vi "Stop Producer LV2.vi"(0 "Stop":bool, 11 "Error In":errorcluster, 13 "Operation":T1) -> (4 "Stop":bool, 15 "Error Out":errorcluster)   [LabVIEW 2023]
doc: "The file is the functional global to store the status of the stop boolean which stops the producer loop."
uses:
  Typedef/User Event Operations.ctl
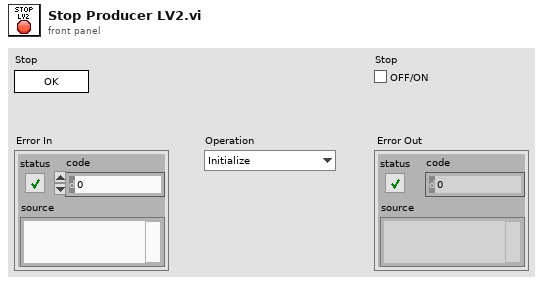
[diagram p1: front panel]
types:
  T1 = typedef "User Event Operations.ctl" = enum16{"Initialize", "Read", "Write"}
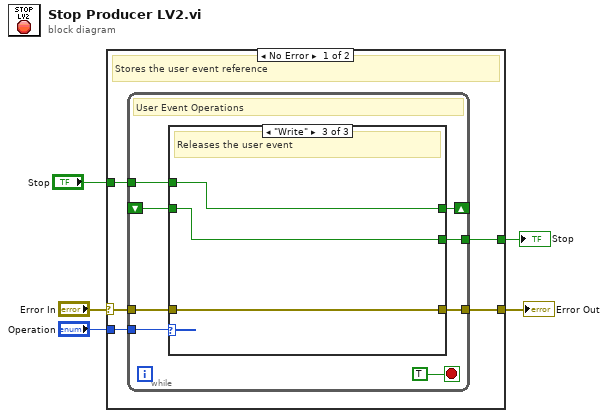
[diagram p0: block diagram]
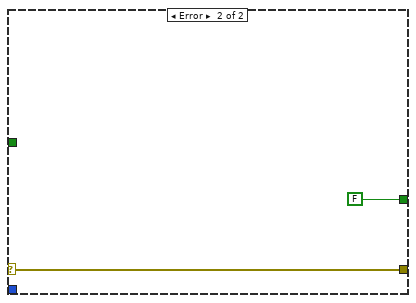
[diagram p4: hidden frame]
diagram:
  n1 = case shown="No Error" "Error In" {
    selector: "Error In" -> [w9 w28]
    tunnel: "Operation" -> [w10 _]
    tunnel: [w8 w28] -> w3
    tunnel: "Stop" -> [w7 _]
    tunnel: [w6 FALSE ("Stop")] -> w1
    frame No Error {
      # "Stores the user event reference"
      n2 = while {
        tunnel: w10 -> [w18]
        tunnel: w9 -> [w17]
        tunnel: [w16] -> w8
        shift-right: [w15] -> _
        shift-left: _ -> [w14]
        tunnel: w7 -> [w12]
        tunnel: [w11] -> w6
        stop <- TRUE stop-if-true
        # "User Event Operations"
        n3 = case shown="\"Write\"" w18 {
          tunnel: w17 -> [w21 w23 w26]
          tunnel: [w21 w23 w26] -> w16
          tunnel: [w20 w22 w25] -> w15
          tunnel: w14 -> [w19 w22 w24]
          tunnel: w12 -> [w20 _ w25]
          tunnel: [w19 w22 w24] -> w11
          frame "Initialize", Default {
            # "Creates or reads the reference"
          }
          frame "Read" {
            # "Generates the user event"
          }
          frame "Write" {
            # "Releases the user event"
          }
        }
      }
    }
    frame Error {
    }
  }
  "Error Out" <- w3
  "Stop" <- w1
